vi "MeasureRMS.vi"(9 "# of Samples":dbl, 10 "Sampling Rate":dbl) -> (1 "Waveform Graph":dynamicdata(graph), 2 "RMS":dbl)   [LabVIEW 2014]
doc: "Measures the voltage on ai 0, and displays the RMS, given a sampling rate and number of samples to take.\n\nBryan Ghahremani - SID: 1135515\nKenneth Heide - SID: 1269429"
uses:
  <vilib>/Analysis/NI_AALPro.lvlib
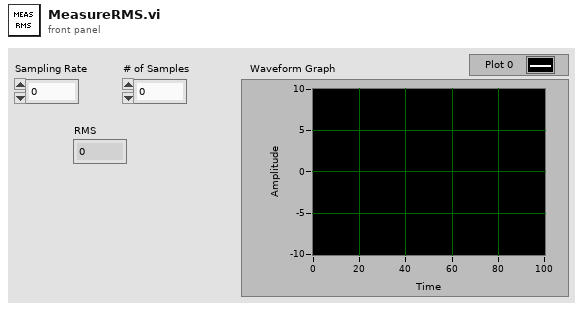
[diagram p1: front panel]
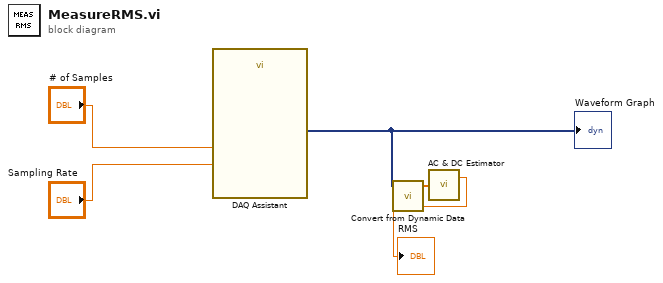
[diagram p0: block diagram]
diagram:
  n1 = call "DAQ Assistant"("rate"="Sampling Rate", "number of samples"="# of Samples") -> ("data"=w3:dynamicdata)  [unwired: 15 in, 2 out]
  "Waveform Graph" <- w3
  n2 = call "Convert from Dynamic Data"("Dynamic Data Type"=w3) -> ("Array"=w2:dbl[])  [unwired: 3 in]
  n3 = call <vilib>:"AC & DC Estimator.vi"("Signal (V)"=w2) -> ("AC estimate (Vrms)"=→"RMS":dbl)  [unwired: 1 out]
